vi "L0_Init.vi"(8 "error in":errorcluster, 11 "connection ID in":refnum<k5>) -> (0 "error out":errorcluster, 3 "connection ID out":refnum<k5>)   [LabVIEW 2009]
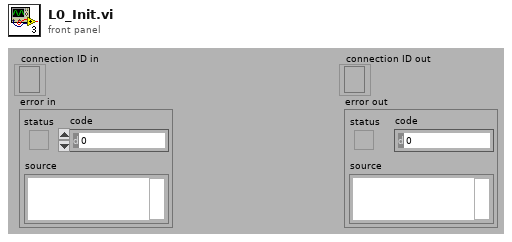
[diagram p1: front panel]
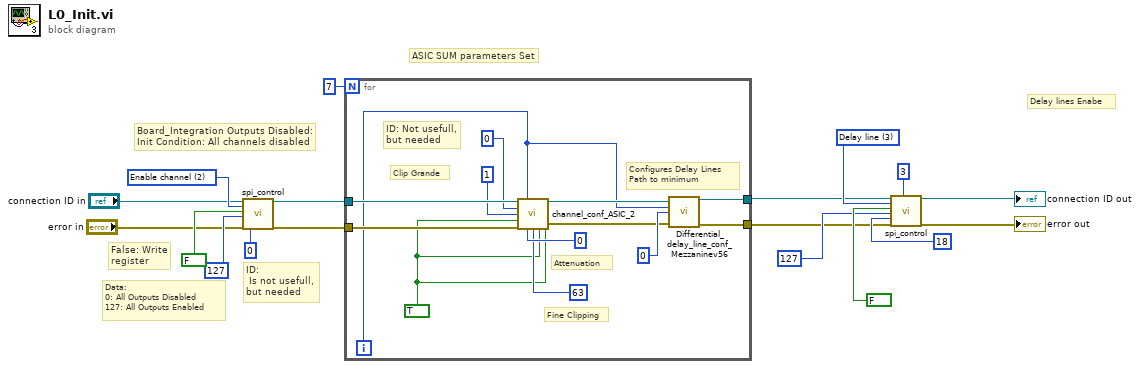
[diagram p0: block diagram]
diagram:
  w6 = u16 3 items=["Attenuation", "Clipping", "Enable channel", "Delay line", "ASIC"] ("Device")
  w17 = u16 2 items=["Attenuation", "Clipping", "Enable channel", "Delay line", "ASIC"] ("Device")
  # "ASIC SUM parameters Set"
  # "False: Write\nregister"
  # "Data:\n0: All Outputs Disabled\n127: All Outputs Enabled"
  # "ID:\n Is not usefull, \nbut needed"
  # "Board_Integration Outputs Disabled:\nInit Condition: All channels disabled"
  # "Delay lines Enabe"
  n1 = call "spi_control.vi"("connection ID"="connection ID in", "Device"=w17, "Read/#write"=FALSE, "Data"=127, "error out 3"="error in", "Id in"=0) -> ("connection ID out"=w11:refnum<k5>, "error out 2"=w10:errorcluster)  [unwired: 6 in, 6 out]
  n2 = for {
    N: 7 -> [_]
    tunnel: w10 -> [w31]
    tunnel: w11 -> [w30]
    tunnel: [w20] -> w4
    tunnel: [w21] -> w3
    i -> [w19]
    w25 = TRUE ("maj/sum")
    # "Configures Delay Lines\nPath to minimum"
    # "Attenuation"
    # "Fine Clipping"
    # "Clip Grande"
    # "ID: Not usefull,\nbut needed"
    n3 = call "channel_conf_ASIC_2.vi"("connection ID"=w30, "Ring"=w19, "Id in"=u32 0, "Clip_sel_b"=u32 1, "CompBuf_en_b"=w25, "error out"=w31, "Att gain"=u32 0, "Ib_ClipVb"=u32 63, "Clip_en_b"=w25, "Att_en_b"=w25) -> ("connection ID out"=w23:refnum<k5>, "error out 2"=w22:errorcluster)  [unwired: 1 in, 3 out]
    n4 = call "Differential_delay_line_conf_Mezzaninev56.vi"("connection ID"=w23, "channel"=w19, "Delay value"=u16 0, "error in (no error)"=w22) -> ("connection ID out"=w20:refnum<k5>, "error out 2"=w21:errorcluster)  [unwired: 4 in, 6 out]
  }
  n5 = call "spi_control.vi"("connection ID"=w4, "Device"=w6, "Read/#write"=FALSE, "Data"=127, "Register or channel"=18, "error out 3"=w3, "chip delay"=3) -> ("connection ID out"=→"connection ID out":refnum<k5>, "error out 2"=→"error out":errorcluster)  [unwired: 5 in, 6 out]
